vi "toml_api_set.vi"(6 "value":variant, 7 "resolved path":path, 8 "error in (no error)":errorcluster, 9 "key":string, 10 "section":string, 11 "vi in":refnum<vi>) -> (0 "error out":errorcluster, 2 "key exists":bool, 3 "vi out":refnum<vi>)   [LabVIEW 2017]
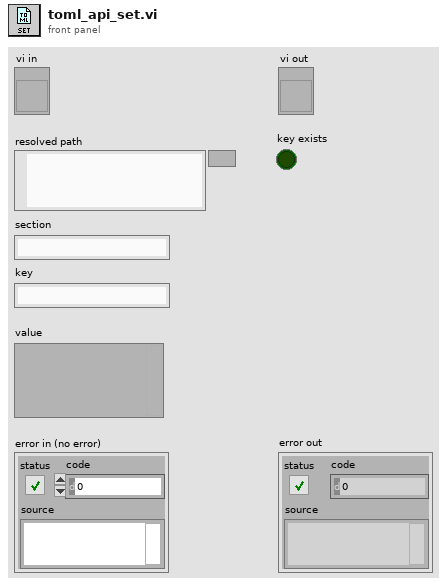
[diagram p1: front panel]
types:
  T1 = cluster{"section":string, "key":string, "default":variant}
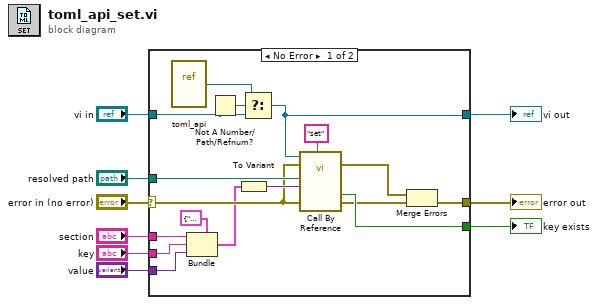
[diagram p0: block diagram]
diagram:
  n1 = case shown="No Error" "error in (no error)" {
    selector: "error in (no error)" -> [w17 w28]
    tunnel: [w25 _] -> w9
    tunnel: "resolved path" -> [w23 _]
    tunnel: [w19 w28] -> w7
    tunnel: "vi in" -> [w16 w27]
    tunnel: [w15 w27] -> w4
    tunnel: "section" -> [w14 _]
    tunnel: "key" -> [w13 _]
    tunnel: "value" -> [w12 _]
    frame No Error {
      n2 = vi-ref "toml_api.vi"() -> (w22:refnum<vi>)
      n3 = Bundle(cluster=T1 {"section"="", "key"="", "default"=variant}, "section"=w14, "key"=w13, "default"=w12) -> (w11:T1)
      n4 = Not A Number/Path/Refnum?(number/path/refnum=w16) -> (NaN/Path/Refnum?=w21:bool)
      n5 = To Variant(anything=w11) -> (Variant=w26:variant)
      n6 = Select(t=w22, s=w21, f=w16) -> (s? t:f=w15:refnum<vi>)
      n7 = call-by-ref "?"(reference=w15, error in=w17, "cmd"="set", 8:"error in (no error)"=w17, "data in"=w26, "path in"=w23) -> (error out=w18:errorcluster, 0:"error out"=w24:errorcluster, "return"=w25:bool)  [unwired: 4 in, 3 out]
      n8 = Merge Errors(w18, w24) -> (w19:errorcluster)
    }
    frame Error {
    }
  }
  "key exists" <- w9
  "error out" <- w7
  "vi out" <- w4
